vi "Name (Local) Taken.vi"(8 "error in (no error)":errorcluster, 10 "Name (Local)":string) -> (0 "error out":errorcluster)   [LabVIEW 2018, in "Application.lvlib" / "Exceptions.lvclass"]
uses:
  Exceptions.lvclass
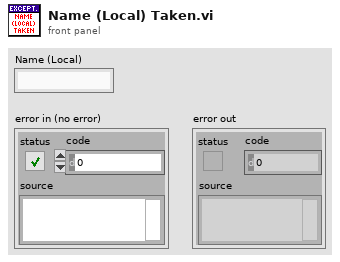
[diagram p1: front panel]
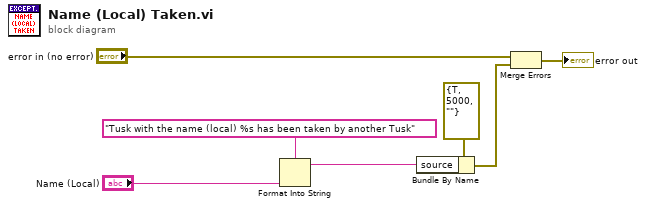
[diagram p0: block diagram]
diagram:
  n1 = Format Into String(format string="Tusk with the name (local) %s has been taken by another Tusk" ("source"), "Name (Local)") -> (resulting string=w6:string)  [unwired: 2 in, 1 out]
  n2 = Bundle By Name(cluster=errorcluster {"status"=TRUE, "code"=5000, "source"=""} ("error out"), "source"=w6) -> (w3:errorcluster)
  n3 = Merge Errors("error in (no error)", w3) -> (→"error out":errorcluster)
